vi "Security.MasterKeyChannelValues.Set.vi"(8 "error in (no error)":errorcluster, 10 "Master Key":string, 11 "Device Item Ref in":T1 format="%.0x") -> (0 "error out":errorcluster, 3 "Section Ref out":T1 format="%.0x")   [LabVIEW 2019, in "Diagnostics Addon System Explorer.lvlib"]
uses:
  Diagnostics Addon System Explorer.lvlib
  <vilib>/NI VeriStand/Custom Device API/Custom Device Item Ref.ctl
  Addon Shared/SubVIs/Constants.vi
  <vilib>/NI VeriStand/Custom Device Tools/Custom Device Utility Library/NI VeriStand - Search for Item by GUID.vi
  <vilib>/NI VeriStand/Custom Device Tools/Custom Device Utility Library/NI VeriStand - Search for Item by Name.vi
  Addon Shared/Diagnostics Addon Shared.lvlib
  <vilib>/NI VeriStand/Custom Device API/Custom Device API.lvlib
  <vilib>/NI VeriStand/Custom Device Tools/Custom Device Utility Library/Custom Device Utility Library.lvlib
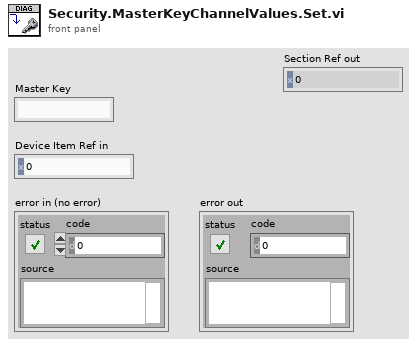
[diagram p1: front panel]
types:
  T1 = typedef "Custom Device API.lvlib/Custom Device Item Ref.ctl" = u64
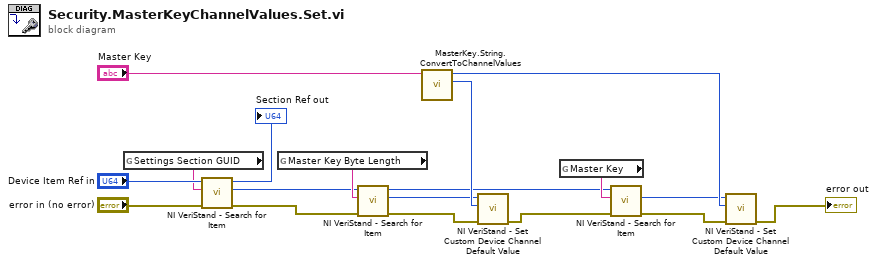
[diagram p0: block diagram]
diagram:
  n1 = global read "Constants.vi" "Settings Section GUID"() -> (w2:string)
  n2 = call-poly <vilib>:"NI VeriStand - Search for Item.vi"("error in"="error in (no error)", "Item GUID"=w2, "Section Ref in"="Device Item Ref in") -> ("error out"=w6:errorcluster, "Item Ref"=w5:T1, "Section Ref out"=→"Section Ref out":T1)  [unwired: 5 in, 1 out]
  n3 = global read "Constants.vi" "Master Key Byte Length"() -> (w7:string)
  n4 = call-poly <vilib>:"NI VeriStand - Search for Item.vi"("error in"=w6, "Item Name"=w7, "Section Ref in"=w5) -> ("error out"=w8:errorcluster, "Item Ref"=w9:T1, "Section Ref out"=w10:T1)  [unwired: 5 in, 1 out]
  n5 = call "MasterKey.String.ConvertToChannelValues.vi"("Master Key"="Master Key") -> ("Length"=w18:i32, "Value"=w17:u64)  [unwired: 9 in]
  n6 = call <vilib>:"NI VeriStand - Set Custom Device Channel Default Value.vi"("error in (no error)"=w8, "Default Value"=w18, "Channel Ref in"=w9) -> ("error out"=w12:errorcluster)  [unwired: 7 in, 1 out]
  n7 = global read "Constants.vi" "Master Key"() -> (w11:string)
  n8 = call-poly <vilib>:"NI VeriStand - Search for Item.vi"("error in"=w12, "Item Name"=w11, "Section Ref in"=w10) -> ("error out"=w14:errorcluster, "Item Ref"=w13:T1)  [unwired: 5 in, 2 out]
  n9 = call <vilib>:"NI VeriStand - Set Custom Device Channel Default Value.vi"("error in (no error)"=w14, "Default Value"=w17, "Channel Ref in"=w13) -> ("error out"=→"error out":errorcluster)  [unwired: 7 in, 1 out]
